vi "Get SMO RC Type.vi"(8 "error in (no error)":errorcluster, 11 "Inst.TCInstrument in":refnum<class "Inst.TC.lvclass">) -> (0 "error out":errorcluster, 2 "RemoteControl":refnum<class "RemoteControl.lvclass">, 3 "Inst.TCInstrument out":refnum<class "Inst.TC.lvclass">)   [LabVIEW 2019, in "Inst.TC.lvclass"]
uses:
  Inst.TC.lvclass
  <userlib>/LevyLab/Instrument Framework/Instrument Types/VSource/Instrument.VSource.lvclass
  <userlib>/LevyLab/RemoteControl/RemoteControl/RemoteControl.lvclass
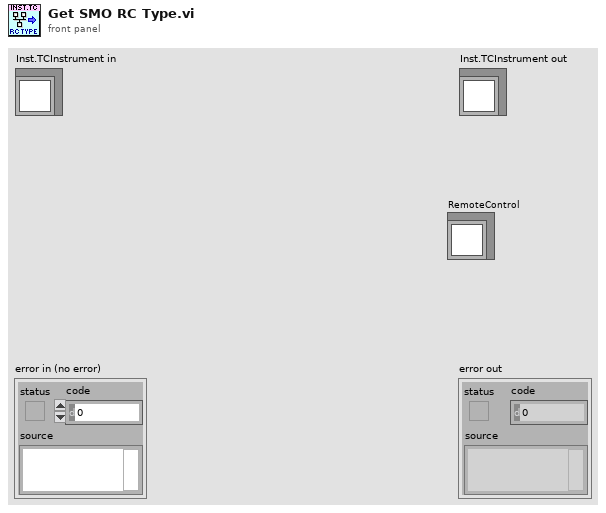
[diagram p1: front panel]
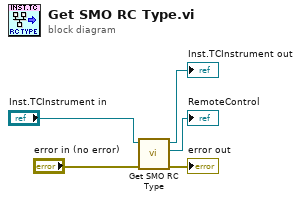
[diagram p0: block diagram]
diagram:
  n1 = call-parent "Get SMO RC Type.vi"("error in (no error)"="error in (no error)", "Instrument in"="Inst.TCInstrument in") -> ("error out"=→"error out":errorcluster, "RemoteControl"=→"RemoteControl":refnum<class "RemoteControl.lvclass">, "Instrument out"=→"Inst.TCInstrument out":refnum<class "Inst.TC.lvclass">)  [unwired: 7 in]
